vi "Start Sync.vi"(8 "error in (no error)":errorcluster, 11 "gRPC Server in":refnum<class "MeasurementService.lvclass">) -> (0 "error out":errorcluster, 3 "gRPC Server out":refnum<class "MeasurementService.lvclass">)   [LabVIEW 2020, in "Load Regulation.lvlib" / "MeasurementService.lvclass"]
uses:
  MeasurementService.lvclass
  MeasurementService.lvclass/MeasurementService.ctl
  5f4d23ba-5f3b-4d21-973a-1787d5e97601.vi
  b60fc25a-b586-4512-9a06-4ef685625b50.vi
  Load Regulation.lvlib
  Measurement Configuration.ctl
  RPC Messages/ni_measurements_v1_MeasurementDetails.ctl
  RPC Messages/ni_measurements_v1_ConfigurationParameter.ctl
  RPC Messages/google_protobuf_Any.ctl
  RPC Messages/ni_measurements_v1_Output.ctl
  RPC Messages/ni_measurements_v1_MeasurementParameters.ctl
  RPC Messages/ni_measurements_v1_UserInterfaceDetails.ctl
  RPC Messages/ni_measurements_v1_GetMetadataResponse.ctl
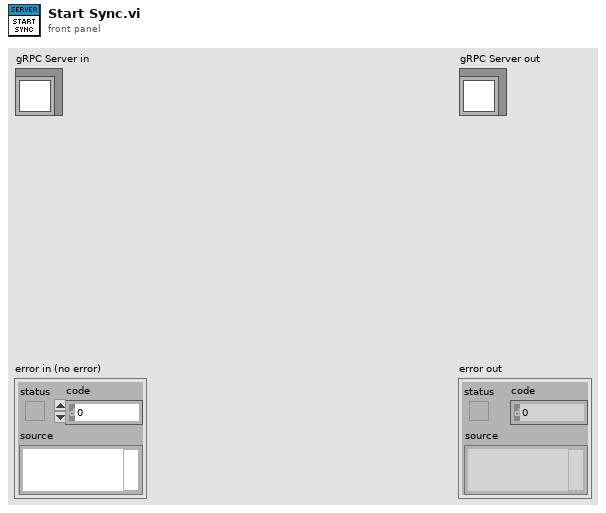
[diagram p1: front panel]
types:
  T1 = typedef "Load Regulation.lvlib/ni_measurements_v1_GetMetadataResponse.ctl" = cluster{"measurement_details":T2, "measurement_parameters":T3, "user_interface_details":T7}
  T2 = typedef "Load Regulation.lvlib/ni_measurements_v1_MeasurementDetails.ctl" = cluster{"display_name":string, "version":string, "measurement_type":string, "product_type":string}
  T3 = typedef "Load Regulation.lvlib/ni_measurements_v1_MeasurementParameters.ctl" = cluster{"configuration_parameters_messagetype":string, "configuration_parameters":T4[], "configuration_defaults":T5, "outputs_message_type":string, "outputs":T6[]}
  T4 = typedef "Load Regulation.lvlib/ni_measurements_v1_ConfigurationParameter.ctl" = cluster{"protobuf_id":u32, "type":i32, "name":string, "repeated":bool}
  T5 = typedef "Load Regulation.lvlib/google_protobuf_Any.ctl" = cluster{"type_url":string, "value":u8[]}
  T6 = typedef "Load Regulation.lvlib/ni_measurements_v1_Output.ctl" = cluster{"protobuf_id":u32, "type":i32, "name":string, "repeated":bool}
  T7 = typedef "Load Regulation.lvlib/ni_measurements_v1_UserInterfaceDetails.ctl" = cluster{"configuration_ui_url":string}
  T8 = typedef "Load Regulation.lvlib/Measurement Configuration.ctl" = cluster{"Input Voltage in V":dbl, "Nominal Output Voltage in V":dbl, "Start":dbl, "Stop":dbl, "Step":dbl, "Input SMU":string, "Load SMU":string, "Input DMM":string, "Load DMM":string}
  T9 = typedef "Load Regulation.lvlib/MeasurementService.lvclass/Server Internal UEs.ctl" = cluster{"ni_measurements_v1_MeasurementService_GetMetadata Internal UE":refnum<user-event>, "ni_measurements_v1_MeasurementService_Measure Internal UE":refnum<user-event>}
  T10 = typedef "Load Regulation.lvlib/MeasurementService.lvclass/Server gRPC UEs.ctl" = cluster{"ni_measurements_v1_MeasurementService_GetMetadata gRPC UE":refnum<user-event>, "ni_measurements_v1_MeasurementService_Measure gRPC UE":refnum<user-event>}
  T11 = typedef "gprc-lvsupport-release.lvlib/grpcId.ctl" = u64
  T12 = typedef "Load Regulation.lvlib/ni_measurements_v1_MeasureRequest.ctl" = cluster{"configuration_parameters":T5}
  T13 = typedef "Load Regulation.lvlib/Measurement Results.ctl" = cluster{"Load Regulation (%)":dbl, "Load Regulation (mV/mA)":dbl, "Test Results.Load Current in A":dbl[], "Output Voltage in V":dbl[]}
  T14 = typedef "gprc-lvsupport-release.lvlib/Any.ctl" = cluster{"Type Url":string, "Bytes":u8[]}
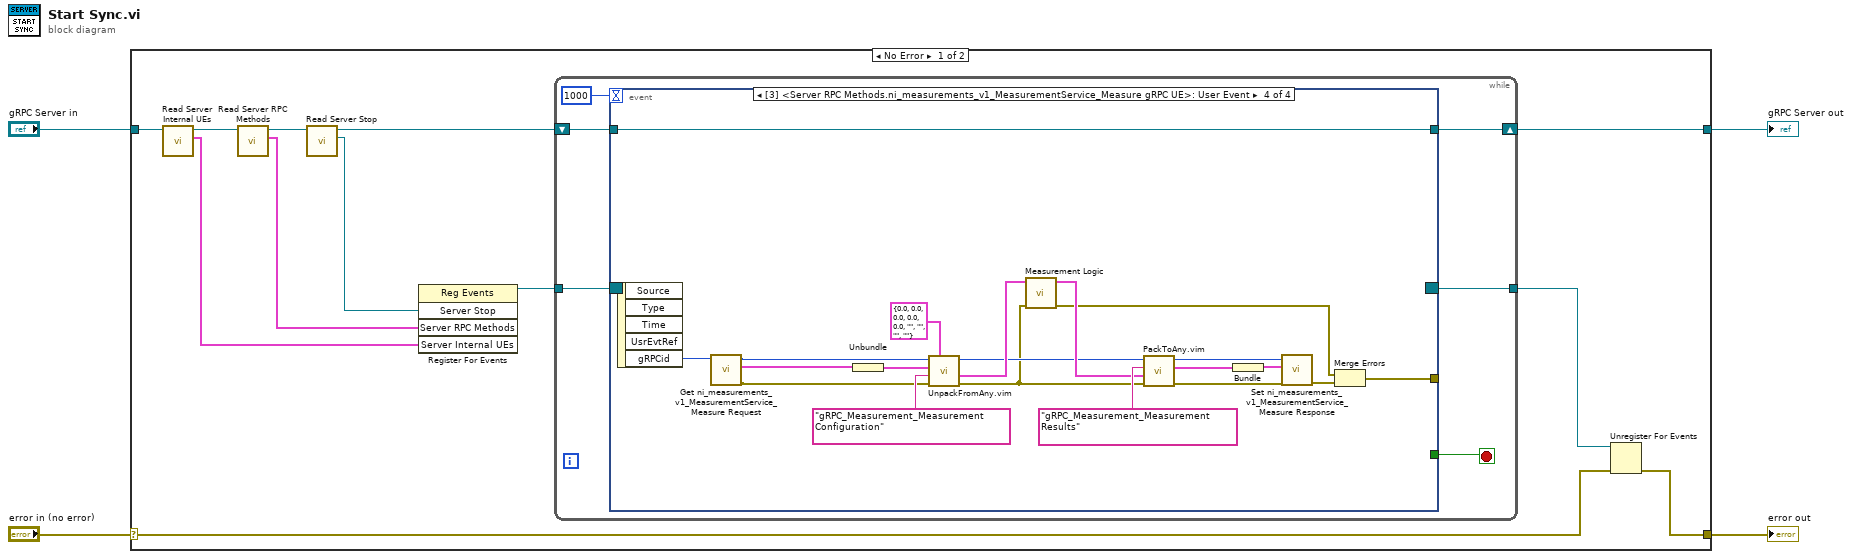
[diagram p0: block diagram]
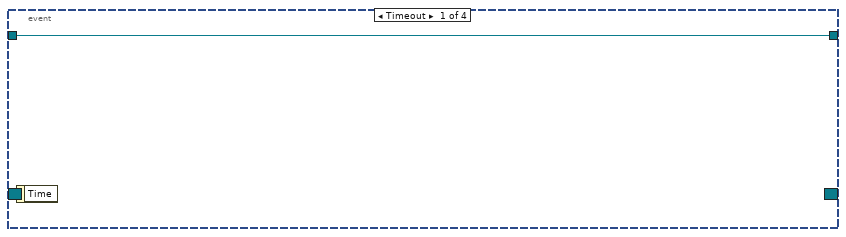
[diagram p2: hidden frame]
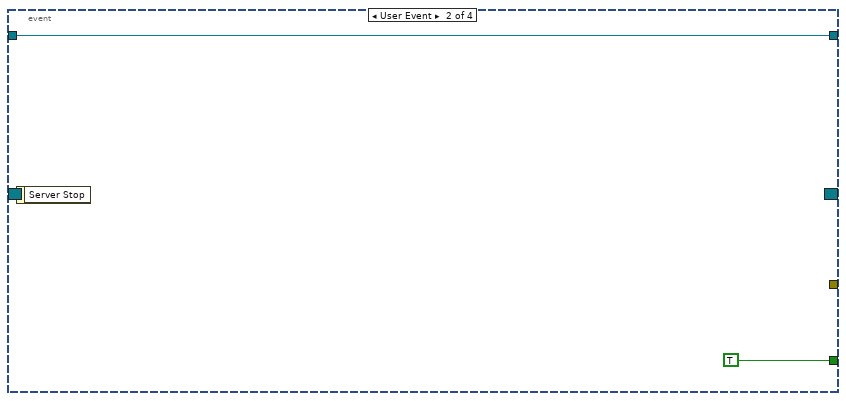
[diagram p3: hidden frame]
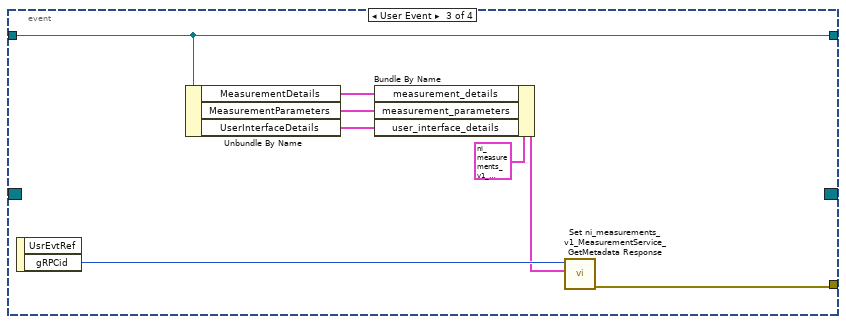
[diagram p4: hidden frame]
diagram:
  n1 = case shown="No Error" "error in (no error)" {
    selector: "error in (no error)" -> [w10 w55]
    tunnel: [w9 w55] -> w3
    tunnel: [w5 w54] -> w1
    tunnel: "gRPC Server in" -> [w16 w54]
    frame No Error {
      n2 = call "Read Server Internal UEs.vi"("SignalGeneratorService in"=w16) -> ("Server Internal UEs"=w14:T9, "SignalGeneratorService out"=w15:refnum<class "MeasurementService.lvclass">)  [unwired: 8 in, 1 out]
      n3 = call "Read Server RPC Methods.vi"("SignalGeneratorService in"=w15) -> ("Server RPC Methods"=w8:T10, "SignalGeneratorService out"=w13:refnum<class "MeasurementService.lvclass">)  [unwired: 8 in, 1 out]
      n4 = call-dynamic "Read Server Stop.vi"("iService in"=w13) -> ("Server Stop"=w7:refnum<user-event>, "iService out"=w6:refnum<class "MeasurementService.lvclass">)  [unwired: 8 in, 1 out]
      n5 = register-events(w7, w8, w14) -> (reference out=w12:refnum<event-registration>)  [unwired: 2 in, 1 out]
      n6 = while {
        tunnel: w12 -> [w22]
        tunnel: [w20] -> w11
        shift-right: [w17] -> w5
        shift-left: w6 -> [w18]
        stop <- w21 stop-if-true
        n7 = event "RPC Methods Event Structure" shown="[3] <Server RPC Methods.ni_measurements_v1_MeasurementService_Measure gRPC UE>: User Event" {
          selector: w22 -> [_ _ _ _]
          dyn-events: [_ _ _ _] -> w20
          timeout: 1000 -> [_ _ _ _]
          tunnel: [_ TRUE _ _] -> w21
          tunnel: [_ _ w31 w35] -> _
          tunnel: w18 -> [w23 w24 w33 w34]
          tunnel: [w23 w24 w33 w34] -> w17
          event Timeout {
            n8 = event-data() -> ()  [unwired: 1 in, 1 out]
          }
          event User Event {
            n9 = event-data() -> ()  [unwired: 1 in, 1 out]
          }
          event User Event {
            n10 = event-data() -> ("gRPCid"=w32:T11)  [unwired: 1 in, 1 out]
            n11 = Unbundle By Name(w33) -> ("MeasurementDetails"=w29:T2, "MeasurementParameters"=w28:T3, "UserInterfaceDetails"=w27:T7)
            n12 = Bundle By Name(cluster=T1 {"measurement_details"={"display_name"="", "version"="", "measurement_type"="", "product_type"=""}, "measurement_parameters"={"configuration_parameters_messagetype"="", "configuration_parameters"=[], "configuration_defaults"={"type_url"="", "value"=[]}, "outputs_message_type"="", "outputs"=[]}, "user_interface_details"={"configuration_ui_url"=""}} ("Message Data"), "measurement_details"=w29, "measurement_parameters"=w28, "user_interface_details"=w27) -> (w26:T1)
            n13 = call "Set ni_measurements_v1_MeasurementService_GetMetadata Response.vi"("Message Data"=w26, "gRPCid in"=w32) -> ("error out"=w31:errorcluster)  [unwired: 9 in]
          }
          event User Event {
            n14 = event-data() -> ("gRPCid"=w45:T11)  [unwired: 1 in, 4 out]
            n15 = call "Get ni_measurements_v1_MeasurementService_Measure Request.vi"("gRPCid in"=w45) -> ("error out"=w43:errorcluster, "Message Data"=w44:T12, "gRPCid out"=w42:T11)  [unwired: 8 in]
            n16 = Unbundle(w44) -> ("configuration_parameters"=w53:T5)
            n17 = call "UnpackFromAny.vim"("Data Type"=T8 {"Input Voltage in V"=0.0, "Nominal Output Voltage in V"=0.0, "Start"=0.0, "Stop"=0.0, "Step"=0.0, "Input SMU"="", "Load SMU"="", "Input DMM"="", "Load DMM"=""} ("Measurement Configuration"), "error in (no error)"=w43, "Message Type"="gRPC_Measurement_Measurement Configuration", "Any"=w53, "gRPCid in"=w42) -> ("error out"=w46:errorcluster, "Unpacked Value"=w49:T8, "gRPCid"=w47:u64)  [unwired: 4 in]
            n18 = call "Measurement Logic.vi"("error in"=w46, "Measurement Configuration"=w49) -> ("error out"=w36:errorcluster, "Measurement Results"=w50:T13)  [unwired: 8 in]
            n19 = call "PackToAny.vim"("error in (no error)"=w46, "Data To Pack"=w50, "Message Type"="gRPC_Measurement_Measurement Results", "gRPCid in"=w47) -> ("error out"=w38:errorcluster, "Any"=w40:T14, "gRPCid"=w41:u64)  [unwired: 5 in]
            n20 = Bundle("Any"=w40) -> (w39:cluster{"Any":T14})  [unwired: 1 in]
            n21 = call "Set ni_measurements_v1_MeasurementService_Measure Response.vi"("error in (no error)"=w38, "Message Data"=w39, "gRPCid in"=w41) -> ("error out"=w37:errorcluster)  [unwired: 8 in]
            n22 = Merge Errors(w36, w37) -> (w35:errorcluster)
          }
        }
      }
      n23 = Unregister For Events(event registration refnum=w11, error in=w10) -> (error out=w9:errorcluster)
    }
    frame Error {
    }
  }
  "error out" <- w3
  "gRPC Server out" <- w1
